vi "exercicio_operacoes_matematicas.vi"() -> ()   [LabVIEW 2020]
panel:
  out "Multiplicacao":dbl
  out "Divisão":dbl format="%#_2g"
  out "Subtracao":dbl
  out "Soma":dbl
  in  "Número B":dbl
  in  "Número A":dbl
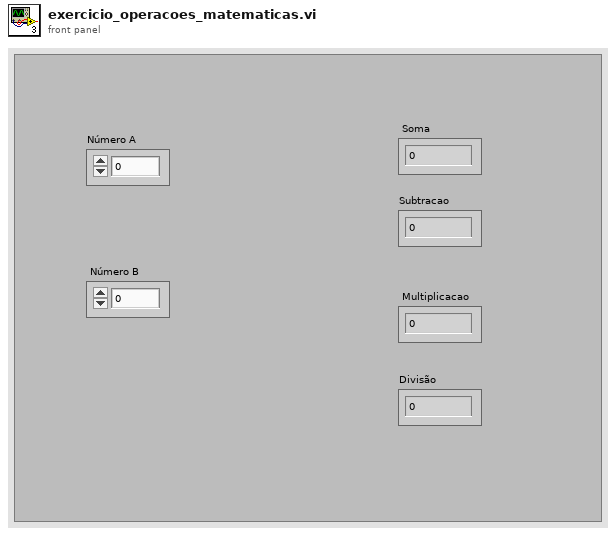
[diagram p1: front panel]
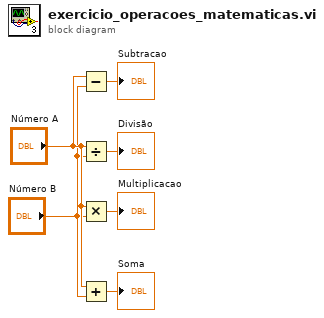
[diagram p0: block diagram]
diagram:
  n1 = Subtract(x="Número A", y="Número B") -> (x-y=→"Subtracao":dbl)
  n2 = Divide(x="Número A", y="Número B") -> (x/y=→"Divisão":dbl)
  n3 = Multiply(x="Número A", y="Número B") -> (x*y=→"Multiplicacao":dbl)
  n4 = Add(x="Número A", y="Número B") -> (x+y=→"Soma":dbl)
